vi "LSMcontroller_v56_from here for labview64bit.vi"() -> ()   [LabVIEW 2015] (continued)
                        n3651 = control-ref of="Digital Lines Plot"() -> (w455:refnum<vi>)
                        n3652 = call "Used DO lines.vi"() -> ("used DO names"=w454:string[], "used DO lines"=w453:tag[])  [unwired: 2 in]
                        n3653 = local write "Analog Used Lines"(w458) -> ()
                        n3654 = local write "Analog Used Names"(w456) -> ()
                        n3655 = local write "Digital Used Lines"(w453) -> ()
                        n3656 = local write "Digital Used Names"(w454) -> ()
                        n3657 = call "prepDOWaveplot.vi"("DigitalGraph in"=w455, "used DO names"=w454) -> ()  [unwired: 1 in]
                        n3658 = call "prepAOWaveplot.vi"("WaveformGraph in"=w457, "Analog Used Names"=w456) -> ()  [unwired: 1 in]
                      }
                    }
                  }
                  frame #4 {
                    n3659 = local read "remAO"() -> (w459:bool)
                    n3660 = case shown="True" w459 {
                      tunnel: w460 -> [_ w461]
                      frame False {
                      }
                      frame True {
                        n3661 = call "waveformparamsv2.vi"("command"="rem AO", "index"=w461) -> ()  [unwired: 3 in, 3 out]
                      }
                    }
                  }
                  frame #5 {
                    n3662 = local read "remAO"() -> (w464:bool)
                    n3663 = case shown="True" w464 {
                      tunnel: w463 -> [_ w483]
                      frame False {
                      }
                      frame True {
                        n3664 = local read "Meastab"() -> (w468:enum32{"X-Y Image", "Linescan", "Timetrace"})
                        n3665 = property on="refwf" class="Ring (strict)"() -> ("RingText.Text"=w471:string)  [unwired: 2 in, 2 out]
                        n3666 = case shown="\"Timetrace\"" w468 {
                          tunnel: [w484 w485] -> w467
                          frame "X-Y Image", Default {
                            n3667 = local read "Sampling rate"() -> (w484:dbl)
                          }
                          frame "Timetrace" {
                            n3668 = local read "srateAODOtt"() -> (w485:dbl)
                          }
                        }
                        n3669 = call "waveformsAObuffer.vi"("command"="get") -> ("AO wf out"=w480:waveform(dbl)[])  [unwired: 1 in]
                        n3670 = call "waveformsDObuffer.vi"("command"="get") -> ("DO wf out"=w477:digitalwaveform[])  [unwired: 1 in]
                        n3671 = Delete From Array(array=w480, length=1, index=w483) -> (array with subset deleted=w472:waveform(dbl)[])  [unwired: 1 out]
                        n3672 = call "correctwaveformsizetemp.vi"("new sampling frequency (Hz)"=w467, "start"=FALSE, "reference waveforms to"=w471, "Analog waveforms in"=w472, "stop"=FALSE, "Digital waveforms in"=w477) -> ("analog wf out"=w475:waveform(dbl)[], "Digital wf out"=w473:digitalwaveform[], "measpoints"=w469:i32)
                        n3673 = local write "Analog Lines Plot"(w475) -> ()
                        n3674 = call "GetNumCamFramesv2.vi"("Digital Waveform Graph"=w473) -> ("Numeric"=w474:i32)  [unwired: 10 in]
                        n3675 = local write "Digital Lines Plot"(w473) -> ()
                        n3676 = call "waveformsAObuffer.vi"("AO wf in"=w475, "command"="set") -> ()  [unwired: 1 out]
                        n3677 = call "waveformsDObuffer.vi"("DO wf in"=w473, "command"="set") -> ()  [unwired: 1 out]
                        n3678 = local read "wavdet"() -> (w470:bool)
                        n3679 = local write "Total Camera Frames"(w474) -> ()
                        n3680 = case shown="True" w470 {
                          tunnel: w469 -> [_ w486]
                          frame False {
                          }
                          frame True {
                            n3681 = local write "# of frames"(w486) -> ()
                          }
                        }
                      }
                    }
                  }
                  frame #6 {
                    w487 = FALSE ("remAO")
                    n3682 = local read "finite samples"() -> (w488:bool)
                    n3683 = local read "continuous"() -> (w489:bool)
                    n3684 = local read "wavdet"() -> (w490:bool)
                    n3685 = call "2pparameters.vi"("command"="get") -> ("params out"=w493:T12)  [unwired: 1 in]
                    n3686 = Bundle By Name(cluster=w493, "finite"=w488, "cont"=w489, "wavdet"=w490) -> (w491:T12)
                    n3687 = local write "remAO"(w487) -> ()
                    n3688 = property on="Rem AO wave" class="Bool (strict)"("Val(Sgnl)"=w487) -> ()  [unwired: 2 in, 2 out]
                    n3689 = call "2pparameters.vi"("Params in"=w491, "command"="set") -> ()  [unwired: 1 out]
                  }
                }
              }
            }
          }
          event "Add DO wave": Value Change {
            n3690 = event-data() -> ("NewVal"=w495:bool)  [unwired: 1 in, 5 out]
            n3691 = case shown="True" w495 {
              frame False {
              }
              frame True {
                n3692 = stacked-sequence {
                  seq-local: [_ _ _ _ _ w655 _ _] -> [_ _ _ _ _ _ w670 _]
                  frame #0 {
                    n3693 = local read "Measurement"() -> (w496:T5)
                    n3694 = case shown="\"X-Y-t movie\", Default" w496 {
                      frame "X-Y-t movie", Default {
                        n3695 = local read "avpp"() -> (w517:i32)
                        n3696 = local read "Angle ref"() -> (w516:dbl)
                        n3697 = local read "ROI Type"() -> (w515:u16)
                        n3698 = local read "xpixels ref"() -> (w512:i32)
                        n3699 = local read "Vx-min ref"() -> (w511:dbl)
                        n3700 = local read "Vx-max ref"() -> (w510:dbl)
                        n3701 = local read "ypixels ref"() -> (w508:i32)
                        n3702 = local read "Vy-min ref"() -> (w509:dbl)
                        n3703 = local read "Vy-max ref"() -> (w505:dbl)
                        n3704 = local read "Sampling rate"() -> (w499:dbl)
                        n3705 = local read "finite samples"() -> (w500:bool)
                        n3706 = local read "continuous"() -> (w503:bool)
                        n3707 = local read "wavdet"() -> (w504:bool)
                        n3708 = local read "# of frames"() -> (w502:i32)
                        n3709 = local read "maxbufferAI"() -> (w501:i32)
                        n3710 = local read "Override AI buffer"() -> (w497:bool)
                        n3711 = call "2pparameters.vi"("command"="get") -> ("params out"=w514:T12)  [unwired: 1 in]
                        n3712 = Bundle By Name(cluster=w514, "type"="X-Y-t movie", "avpp"=w517, "Angle Img"=w516, "Xpixels Img"=w512, "Vx-min Img"=w511, "VX-max Img"=w510, "Ypixels Img"=w508, "Vy-min Img"=w509, "Vy-max Img"=w505, "srate"=w499, "srate Img"=w499, "finite"=w500, "cont"=w503, "wavdet"=w504, "measpoints"=w502, "maxbufferAI"=w501, "Drawing Mode"=w515, "Vz-reset"=0.0, "AIoverride"=w497) -> (w506:T12)
                        n3713 = call "2pparameters.vi"("Params in"=w506, "command"="set") -> ()  [unwired: 1 out]
                      }
                      frame "X-Y-Z stack" {
                        n3714 = call "2pparameters.vi"("command"="get") -> ("params out"=w521:T12)  [unwired: 1 in]
                        n3715 = Bundle By Name(cluster=w521, "type"="X-Y-Z stack") -> (w519:T12)
                        n3716 = call "2pparameters.vi"("Params in"=w519, "command"="set") -> ()  [unwired: 1 out]
                      }
                      frame "Lifetime (scan)" {
                        n3717 = call "2pparameters.vi"("command"="get") -> ("params out"=w526:T12)  [unwired: 1 in]
                        n3718 = Bundle By Name(cluster=w526, "type"="Lifetime (scan)") -> (w524:T12)
                        n3719 = call "2pparameters.vi"("Params in"=w524, "command"="set") -> ()  [unwired: 1 out]
                      }
                      frame "Lifetime (contour)" {
                        n3720 = local read "Vy-min draw"() -> (w536:dbl)
                        n3721 = local read "Vy-max draw"() -> (w535:dbl)
                        n3722 = local read "Vx-min draw"() -> (w538:dbl)
                        n3723 = local read "Vx-max draw"() -> (w537:dbl)
                        n3724 = local read "xpixels ref"() -> (w534:i32)
                        n3725 = local read "ypixels ref"() -> (w533:i32)
                        n3726 = local read "ROI Type"() -> (w532:u16)
                        n3727 = local read "srateAODOtt"() -> (w543:dbl)
                        n3728 = local read "# of frames"() -> (w548:i32)
                        n3729 = local read "refreshtime"() -> (w540:dbl)
                        n3730 = local read "Pel"() -> (w531:dbl)
                        n3731 = local read "bin"() -> (w546:dbl)
                        n3732 = local read "Override AI buffer"() -> (w529:bool)
                        n3733 = local read "finite samples"() -> (w555:bool)
                        n3734 = local read "srateAODOtt"() -> (w542:dbl)
                        n3735 = local read "srateAODOtt"() -> (w549:dbl)
                        n3736 = local read "continuous"() -> (w554:bool)
                        n3737 = local read "Angle ref"() -> (w539:dbl)
                        n3738 = local read "wavdet"() -> (w556:bool)
                        n3739 = local read "Vx-ref"() -> (w551:dbl)
                        n3740 = local read "Vy-ref"() -> (w553:dbl)
                        n3741 = local read "avpp"() -> (w552:i32)
                        n3742 = call "tt_timeandsamples.vi"("bin"=w546, "refreshtime"=w540, "srateAODOtt"=w543, "tot#ofsamples"=w548) -> ("refreshrate"=w544:dbl, "refreshbuffer"=w545:i32, "timetracecycles"=w550:i32)  [unwired: 5 in]
                        n3743 = local read "bin"() -> (w547:dbl)
                        n3744 = call "2pparameters.vi"("command"="get") -> ("params out"=w559:T12)  [unwired: 1 in]
                        n3745 = Bundle By Name(cluster=w559, "Drawing Mode"=w532, "measpoints"=w548, "tt_cycles"=w550, "refreshbuffer"=w545, "refreshrate"=w544, "Vx-ref"=w551, "Vy-ref"=w553, "srate"=w542, "finite"=w555, "cont"=w554, "wavdet"=w556, "avpp"=w552, "srateAODO"=w549, "bufferAI"=w545, "bin"=w547, "Angle Img"=w539, "Vxminref"=w538, "Vxmaxref"=w537, "Vyminref"=w536, "Vymaxref"=w535, "Xpixels Img"=w534, "Ypixels Img"=w533, "Pel"=w531, "Vz-reset"=0.0, "AIoverride"=w529, "type"="Lifetime (contour)") -> (w557:T12)
                        n3746 = Reciprocal(x=w544) -> (1/x=w541:dbl)
                        n3747 = local write "refreshtime"(w541) -> ()
                        n3748 = call "2pparameters.vi"("Params in"=w557, "command"="set") -> ()  [unwired: 1 out]
                      }
                      frame "X-Y-Z-t movie" {
                      }
                      frame "linescan" {
                      }
                      frame "Timetrace" {
                        n3749 = local read "Vy-min draw"() -> (w569:dbl)
                        n3750 = local read "Vy-max draw"() -> (w568:dbl)
                        n3751 = local read "Vx-min draw"() -> (w571:dbl)
                        n3752 = local read "Vx-max draw"() -> (w570:dbl)
                        n3753 = local read "xpixels ref"() -> (w567:i32)
                        n3754 = local read "ypixels ref"() -> (w566:i32)
                        n3755 = local read "ROI Type"() -> (w565:u16)
                        n3756 = local read "srateAODOtt"() -> (w576:dbl)
                        n3757 = local read "# of frames"() -> (w581:i32)
                        n3758 = local read "refreshtime"() -> (w573:dbl)
                        n3759 = local read "Pel"() -> (w564:dbl)
                        n3760 = local read "bin"() -> (w579:dbl)
                        n3761 = local read "Override AI buffer"() -> (w562:bool)
                        n3762 = local read "finite samples"() -> (w588:bool)
                        n3763 = local read "srateAODOtt"() -> (w575:dbl)
                        n3764 = local read "srateAODOtt"() -> (w582:dbl)
                        n3765 = local read "continuous"() -> (w587:bool)
                        n3766 = local read "Angle ref"() -> (w572:dbl)
                        n3767 = local read "wavdet"() -> (w589:bool)
                        n3768 = local read "Vx-ref"() -> (w584:dbl)
                        n3769 = local read "Vy-ref"() -> (w586:dbl)
                        n3770 = local read "avpp"() -> (w585:i32)
                        n3771 = call "tt_timeandsamples.vi"("bin"=w579, "refreshtime"=w573, "srateAODOtt"=w576, "tot#ofsamples"=w581) -> ("refreshrate"=w577:dbl, "refreshbuffer"=w578:i32, "timetracecycles"=w583:i32)  [unwired: 5 in]
                        n3772 = local read "bin"() -> (w580:dbl)
                        n3773 = call "2pparameters.vi"("command"="get") -> ("params out"=w592:T12)  [unwired: 1 in]
                        n3774 = Bundle By Name(cluster=w592, "Drawing Mode"=w565, "measpoints"=w581, "tt_cycles"=w583, "refreshbuffer"=w578, "refreshrate"=w577, "Vx-ref"=w584, "Vy-ref"=w586, "srate"=w575, "finite"=w588, "cont"=w587, "wavdet"=w589, "avpp"=w585, "srateAODO"=w582, "bufferAI"=w578, "bin"=w580, "Angle Img"=w572, "Vxminref"=w571, "Vxmaxref"=w570, "Vyminref"=w569, "Vymaxref"=w568, "Xpixels Img"=w567, "Ypixels Img"=w566, "Pel"=w564, "Vz-reset"=0.0, "AIoverride"=w562, "type"="Timetrace") -> (w590:T12)
                        n3775 = Reciprocal(x=w577) -> (1/x=w574:dbl)
                        n3776 = local write "refreshtime"(w574) -> ()
                        n3777 = call "2pparameters.vi"("Params in"=w590, "command"="set") -> ()  [unwired: 1 out]
                      }
                      frame "Lifetime (point)" {
                      }
                    }
                  }
                  frame #1 {
                    w595 = FALSE ("wavdet")
                    n3778 = call "2pparameters.vi"("command"="get") -> ("params out"=w599:T12)  [unwired: 1 in]
                    n3779 = Bundle By Name(cluster=w599, "finite"=w595, "cont"=w595, "wavdet"=TRUE) -> (w596:T12)
                    n3780 = call "2pparameters.vi"("Params in"=w596, "command"="set") -> ()  [unwired: 1 out]
                  }
                  frame #2 {
                    n3781 = local read "DO channels"() -> (w606:u16)
                    n3782 = call "2pparameters.vi"("command"="get") -> ("params out"=w604:T12)  [unwired: 1 in]
                    n3783 = in-place {
                      in-place-border: w606 -> [w610]
                      in-place-border: [w607] -> w601
                      n3784 = in-place-cluster #51(w604) -> ("aDO"=w609:u32[])
                      n3785 = call "add channel to active arrayv2.vi"("line array in"=w609, "line to add"=w610) -> ("line array out"=w608:u32[], "addition"=w607:bool)  [unwired: 1 out]
                      n3786 = in-place-cluster #51("aDO"=w608) -> (w602:T12)
                    }
                    n3787 = local write "addDO"(w601) -> ()
                    n3788 = call "2pparameters.vi"("Params in"=w602, "command"="set") -> ()  [unwired: 1 out]
                  }
                  frame #3 {
                    n3789 = local read "addDO"() -> (w611:bool)
                    n3790 = case shown="True" w611 {
                      frame False {
                      }
                      frame True {
                        n3791 = call "Used AO lines.vi"() -> ("used AO names"=w615:string[], "used AO lines"=w617:tag[])  [unwired: 2 in]
                        n3792 = control-ref of="Analog Lines Plot"() -> (w616:refnum<vi>)
                        n3793 = control-ref of="Digital Lines Plot"() -> (w614:refnum<vi>)
                        n3794 = call "Used DO lines.vi"() -> ("used DO names"=w613:string[], "used DO lines"=w612:tag[])  [unwired: 2 in]
                        n3795 = local write "Analog Used Lines"(w617) -> ()
                        n3796 = local write "Analog Used Names"(w615) -> ()
                        n3797 = local write "Digital Used Lines"(w612) -> ()
                        n3798 = local write "Digital Used Names"(w613) -> ()
                        n3799 = call "prepDOWaveplot.vi"("DigitalGraph in"=w614, "used DO names"=w613) -> ()  [unwired: 1 in]
                        n3800 = call "prepAOWaveplot.vi"("WaveformGraph in"=w616, "Analog Used Names"=w615) -> ()  [unwired: 1 in]
                      }
                    }
                  }
                  frame #4 {
                    n3801 = local read "addDO"() -> (w618:bool)
                    n3802 = case shown="True" w618 {
                      frame False {
                      }
                      frame True {
                        n3803 = local read "Build digital waveform tabs"() -> (w619:enum32{"Simple", "Matlab"})
                        n3804 = case shown="\"Matlab\"" w619 {
                          frame "Simple", Default {
                            n3805 = local read "Meastab"() -> (w621:enum32{"X-Y Image", "Linescan", "Timetrace"})
                            n3806 = call "waveformparamsv2.vi"("command"="get") -> ("Params out"=w635:T16)  [unwired: 4 in, 2 out]
                            n3807 = case shown="\"Timetrace\"" w621 {
                              tunnel: [w637 w638] -> w620
                              frame "X-Y Image", Default {
                                n3808 = local read "Sampling rate"() -> (w637:dbl)
                              }
                              frame "Timetrace" {
                                n3809 = local read "srateAODOtt"() -> (w638:dbl)
                              }
                            }
                            n3810 = Unbundle By Name(w635) -> ("DO parameters"=w633:T19)
                            n3811 = local read "Digital padding value"() -> (w624:dbl)
                            n3812 = local read "Digital time offset (s)"() -> (w625:dbl)
                            n3813 = local read "Digital phase (s)"() -> (w627:dbl)
                            n3814 = local read "Digital Freq (Hz)"() -> (w626:dbl)
                            n3815 = local read "Digital DC (%)"() -> (w628:dbl)
                            n3816 = Index Array(array=w633, index=0) -> (element=w632:T20)
                            n3817 = Bundle By Name(cluster=w632, "Digital DC (%)"=w628, "Digital phase"=w627, "Digital Freq (Hz)"=w626, "Sampling frequency (Hz)"=w620, "Digital time offset (s)"=w625, "padding value"=w624, "matlab wave file"=path "", "DOtab"=0.0) -> (w630:T20)
                            n3818 = Build Array(w630) -> (w629:T19)
                            n3819 = call "waveformparamsv2.vi"("command"="add DO", "add DO"=w629) -> ()  [unwired: 3 in, 3 out]
                          }
                          frame "Matlab" {
                            w642 = 0.0 ("DOtab")
                            n3820 = local read "Meastab"() -> (w640:enum32{"X-Y Image", "Linescan", "Timetrace"})
                            n3821 = call "waveformparamsv2.vi"("command"="get") -> ("Params out"=w651:T16)  [unwired: 4 in, 2 out]
                            n3822 = case shown="\"Timetrace\"" w640 {
                              tunnel: [w653 w654] -> w639
                              frame "X-Y Image", Default {
                                n3823 = local read "Sampling rate"() -> (w653:dbl)
                              }
                              frame "Timetrace" {
                                n3824 = local read "srateAODOtt"() -> (w654:dbl)
                              }
                            }
                            n3825 = Unbundle By Name(w651) -> ("DO parameters"=w649:T19)
                            n3826 = local read "Matlab waveform path DO"() -> (w641:path)
                            n3827 = local read "Matlab padding value DO"() -> (w644:dbl)
                            n3828 = Index Array(array=w649, index=0) -> (element=w648:T20)
                            n3829 = Bundle By Name(cluster=w648, "Digital DC (%)"=w642, "Digital phase"=w642, "Digital Freq (Hz)"=w642, "Sampling frequency (Hz)"=w639, "Digital time offset (s)"=w642, "padding value"=w644, "matlab wave file"=w641, "DOtab"=1.0) -> (w646:T20)
                            n3830 = Build Array(w646) -> (w645:T19)
                            n3831 = call "waveformparamsv2.vi"("command"="add DO", "add DO"=w645) -> ()  [unwired: 3 in, 3 out]
                          }
                        }
                      }
                    }
                  }
                  frame #5 {
                    n3832 = local read "addDO"() -> (w656:bool)
                    n3833 = case shown="True" w656 {
                      tunnel: [_ w657] -> w655
                      frame False {
                      }
                      frame True {
                        n3834 = property on="refwf" class="Ring (strict)"() -> ("RingText.Text"=w662:string)  [unwired: 2 in, 2 out]
                        n3835 = call "waveformsDObuffer.vi"("command"="get") -> ("DO wf out"=w661:digitalwaveform[])  [unwired: 1 in]
                        n3836 = call "waveformsAObuffer.vi"("command"="get") -> ("AO wf out"=w659:waveform(dbl)[])  [unwired: 1 in]
                        n3837 = call "referfencesize.vi"("Digital waveforms in"=w661, "Analog waveforms in"=w659, "reference waveforms to"=w662) -> ("number of samples"=w657:i32)  [unwired: 2 in]
                      }
                    }
                  }
                  frame #6 {
                    n3838 = local read "Build digital waveform tabs"() -> (w673:enum32{"Simple", "Matlab"})
                    n3839 = call "waveformparamsv2.vi"("command"="get last DO") -> ("last DO"=w672:T20)  [unwired: 4 in, 2 out]
                    n3840 = local read "Meastab"() -> (w666:enum32{"X-Y Image", "Linescan", "Timetrace"})
                    n3841 = call "waveformsDObuffer.vi"("command"="get") -> ("DO wf out"=w671:digitalwaveform[])  [unwired: 1 in]
                    n3842 = case shown="\"Simple\", Default" w673 {
                      tunnel: w672 -> [w690 w692]
                      tunnel: w670 -> [w689 _]
                      tunnel: [w688 w691] -> w669
                      frame "Simple", Default {
                        n3843 = call "simple digital from wf params.vi"("waveform params"=w690, "number of samples"=w689) -> ("digital waveform"=w688:digitalwaveform)
                      }
                      frame "Matlab" {
                        n3844 = call "matlabDOwffromparam.vi"("waveform params"=w692) -> ("digital waveform"=w691:digitalwaveform)
                      }
                    }
                    n3845 = property on="refwf" class="Ring (strict)"() -> ("RingText.Text"=w676:string)  [unwired: 2 in, 2 out]
                    n3846 = case shown="\"Timetrace\"" w666 {
                      tunnel: [w685 w686] -> w665
                      frame "X-Y Image", Default {
                        n3847 = local read "Sampling rate"() -> (w685:dbl)
                      }
                      frame "Timetrace" {
                        n3848 = local read "srateAODOtt"() -> (w686:dbl)
                      }
                    }
                    n3849 = call "waveformsAObuffer.vi"("command"="get") -> ("AO wf out"=w684:waveform(dbl)[])  [unwired: 1 in]
                    n3850 = Build Array (concatenate)(w671, w669) -> (w675:digitalwaveform[])
                    n3851 = call "correctwaveformsizetemp.vi"("new sampling frequency (Hz)"=w665, "start"=FALSE, "reference waveforms to"=w676, "Analog waveforms in"=w684, "stop"=FALSE, "Digital waveforms in"=w675) -> ("analog wf out"=w679:waveform(dbl)[], "Digital wf out"=w677:digitalwaveform[], "measpoints"=w667:i32)
                    n3852 = local write "Analog Lines Plot"(w679) -> ()
                    n3853 = call "GetNumCamFramesv2.vi"("Digital Waveform Graph"=w677) -> ("Numeric"=w678:i32)  [unwired: 10 in]
                    n3854 = local write "Digital Lines Plot"(w677) -> ()
                    n3855 = call "waveformsAObuffer.vi"("AO wf in"=w679, "command"="set") -> ()  [unwired: 1 out]
                    n3856 = call "waveformsDObuffer.vi"("DO wf in"=w677, "command"="set") -> ()  [unwired: 1 out]
                    n3857 = local write "Total Camera Frames"(w678) -> ()
                    n3858 = local read "wavdet"() -> (w668:bool)
                    n3859 = case shown="True" w668 {
                      tunnel: w667 -> [_ w687]
                      frame False {
                      }
                      frame True {
                        n3860 = local write "# of frames"(w687) -> ()
                      }
                    }
                  }
                  frame #7 {
                    w693 = FALSE ("addAO")
                    n3861 = local read "finite samples"() -> (w694:bool)
                    n3862 = local read "continuous"() -> (w695:bool)
                    n3863 = local read "wavdet"() -> (w696:bool)
                    n3864 = call "2pparameters.vi"("command"="get") -> ("params out"=w699:T12)  [unwired: 1 in]
                    n3865 = Bundle By Name(cluster=w699, "finite"=w694, "cont"=w695, "wavdet"=w696) -> (w697:T12)
                    n3866 = call "2pparameters.vi"("Params in"=w697, "command"="set") -> ()  [unwired: 1 out]
                    n3867 = local write "addDO"(w693) -> ()
                    n3868 = property on="Add DO wave" class="Bool (strict)"("Val(Sgnl)"=w693) -> ()  [unwired: 2 in, 2 out]
                  }
                }
              }
            }
          }
          event "DO channels": Value Change {
            n3869 = event-data() -> ()  [unwired: 1 in, 6 out]
            n3870 = local read "DO channels"() -> (w703:u16)
            n3871 = call "2pparameters.vi"("command"="get") -> ("params out"=w705:T12)  [unwired: 1 in]
            n3872 = Unbundle By Name(w705) -> ("aDO"=w704:u32[])
            n3873 = Search 1D Array(1D array=w704, element=w703) -> (index of element=w702:i32)  [unwired: 1 in]
            n3874 = Equal?(x=w702, y=-1.0) -> (x = y?=w701:bool)
            n3875 = case shown="False" w701 {
              tunnel: w702 -> [w720 _]
              frame False {
                n3876 = call "waveformparamsv2.vi"("command"="get") -> ("Params out"=w715:T16)  [unwired: 4 in, 2 out]
                n3877 = Unbundle By Name(w715) -> ("DO parameters"=w713:T19)
                n3878 = Index Array(array=w713, index=w720) -> (element=w719:T20)
                n3879 = Unbundle By Name(w719) -> ("Digital DC (%)"=w718:dbl, "Digital phase"=w717:dbl, "Digital Freq (Hz)"=w716:dbl, "Sampling frequency (Hz)"=w708:dbl, "Digital time offset (s)"=w712:dbl, "padding value"=w711:dbl, "matlab wave file"=w710:path, "DOtab"=w709:dbl)
                n3880 = local write "Build digital waveform tabs"(w709) -> ()
                n3881 = local write "Digital DC (%)"(w718) -> ()
                n3882 = local write "Matlab waveform path DO"(w710) -> ()
                n3883 = local write "Digital time offset (s)"(w712) -> ()
                n3884 = local write "Matlab padding value DO"(w711) -> ()
                n3885 = local write "Digital padding value"(w711) -> ()
                n3886 = local write "Sampling rate \ncurrent wf"(w708) -> ()
                n3887 = local write "Digital Freq (Hz)"(w716) -> ()
                n3888 = local write "Digital phase (s)"(w717) -> ()
              }
              frame True {
              }
            }
          }
          event "Rem DO wave": Value Change {
            n3889 = event-data() -> ("NewVal"=w721:bool)  [unwired: 1 in, 5 out]
            n3890 = case shown="True" w721 {
              frame False {
              }
              frame True {
                n3891 = stacked-sequence {
                  seq-local: [_ _ w827 _ _ _ _] -> [_ _ _ _ w846 w857 _]
                  frame #0 {
                    n3892 = local read "Measurement"() -> (w722:T5)
                    n3893 = case shown="\"linescan\"" w722 {
                      frame "X-Y-t movie", Default {
                        n3894 = local read "avpp"() -> (w743:i32)
                        n3895 = local read "Angle ref"() -> (w742:dbl)
                        n3896 = local read "ROI Type"() -> (w741:u16)
                        n3897 = local read "xpixels ref"() -> (w738:i32)
                        n3898 = local read "Vx-min ref"() -> (w737:dbl)
                        n3899 = local read "Vx-max ref"() -> (w736:dbl)
                        n3900 = local read "ypixels ref"() -> (w734:i32)
                        n3901 = local read "Vy-min ref"() -> (w735:dbl)
                        n3902 = local read "Vy-max ref"() -> (w731:dbl)
                        n3903 = local read "Sampling rate"() -> (w725:dbl)
                        n3904 = local read "finite samples"() -> (w726:bool)
                        n3905 = local read "continuous"() -> (w729:bool)
                        n3906 = local read "wavdet"() -> (w730:bool)
                        n3907 = local read "# of frames"() -> (w728:i32)
                        n3908 = local read "maxbufferAI"() -> (w727:i32)
                        n3909 = local read "Override AI buffer"() -> (w723:bool)
                        n3910 = call "2pparameters.vi"("command"="get") -> ("params out"=w740:T12)  [unwired: 1 in]
                        n3911 = Bundle By Name(cluster=w740, "type"="X-Y-t movie", "avpp"=w743, "Angle Img"=w742, "Xpixels Img"=w738, "Vx-min Img"=w737, "VX-max Img"=w736, "Ypixels Img"=w734, "Vy-min Img"=w735, "Vy-max Img"=w731, "srate"=w725, "srate Img"=w725, "finite"=w726, "cont"=w729, "wavdet"=w730, "measpoints"=w728, "maxbufferAI"=w727, "Drawing Mode"=w741, "Vz-reset"=0.0, "AIoverride"=w723) -> (w732:T12)
                        n3912 = call "2pparameters.vi"("Params in"=w732, "command"="set") -> ()  [unwired: 1 out]
                      }
                      frame "X-Y-Z stack" {
                        n3913 = call "2pparameters.vi"("command"="get") -> ("params out"=w747:T12)  [unwired: 1 in]
                        n3914 = Bundle By Name(cluster=w747, "type"="X-Y-Z stack") -> (w745:T12)
                        n3915 = call "2pparameters.vi"("Params in"=w745, "command"="set") -> ()  [unwired: 1 out]
                      }
                      frame "Lifetime (scan)" {
                        n3916 = call "2pparameters.vi"("command"="get") -> ("params out"=w752:T12)  [unwired: 1 in]
                        n3917 = Bundle By Name(cluster=w752, "type"="Lifetime (scan)") -> (w750:T12)
                        n3918 = call "2pparameters.vi"("Params in"=w750, "command"="set") -> ()  [unwired: 1 out]
                      }
                      frame "Lifetime (contour)" {
                        n3919 = local read "Vy-min draw"() -> (w762:dbl)
                        n3920 = local read "Vy-max draw"() -> (w761:dbl)
                        n3921 = local read "Vx-min draw"() -> (w764:dbl)
                        n3922 = local read "Vx-max draw"() -> (w763:dbl)
                        n3923 = local read "xpixels ref"() -> (w760:i32)
                        n3924 = local read "ypixels ref"() -> (w759:i32)
                        n3925 = local read "ROI Type"() -> (w758:u16)
                        n3926 = local read "srateAODOtt"() -> (w769:dbl)
                        n3927 = local read "# of frames"() -> (w774:i32)
                        n3928 = local read "refreshtime"() -> (w766:dbl)
                        n3929 = local read "Pel"() -> (w757:dbl)
                        n3930 = local read "bin"() -> (w772:dbl)
                        n3931 = local read "Override AI buffer"() -> (w755:bool)
                        n3932 = local read "finite samples"() -> (w781:bool)
                        n3933 = local read "srateAODOtt"() -> (w768:dbl)
                        n3934 = local read "srateAODOtt"() -> (w775:dbl)
                        n3935 = local read "continuous"() -> (w780:bool)
                        n3936 = local read "Angle ref"() -> (w765:dbl)
                        n3937 = local read "wavdet"() -> (w782:bool)
                        n3938 = local read "Vx-ref"() -> (w777:dbl)
                        n3939 = local read "Vy-ref"() -> (w779:dbl)
                        n3940 = local read "avpp"() -> (w778:i32)
                        n3941 = call "tt_timeandsamples.vi"("bin"=w772, "refreshtime"=w766, "srateAODOtt"=w769, "tot#ofsamples"=w774) -> ("refreshrate"=w770:dbl, "refreshbuffer"=w771:i32, "timetracecycles"=w776:i32)  [unwired: 5 in]
                        n3942 = local read "bin"() -> (w773:dbl)
                        n3943 = call "2pparameters.vi"("command"="get") -> ("params out"=w785:T12)  [unwired: 1 in]
                        n3944 = Bundle By Name(cluster=w785, "Drawing Mode"=w758, "measpoints"=w774, "tt_cycles"=w776, "refreshbuffer"=w771, "refreshrate"=w770, "Vx-ref"=w777, "Vy-ref"=w779, "srate"=w768, "finite"=w781, "cont"=w780, "wavdet"=w782, "avpp"=w778, "srateAODO"=w775, "bufferAI"=w771, "bin"=w773, "Angle Img"=w765, "Vxminref"=w764, "Vxmaxref"=w763, "Vyminref"=w762, "Vymaxref"=w761, "Xpixels Img"=w760, "Ypixels Img"=w759, "Pel"=w757, "Vz-reset"=0.0, "AIoverride"=w755, "type"="Lifetime (contour)") -> (w783:T12)
                        n3945 = Reciprocal(x=w770) -> (1/x=w767:dbl)
                        n3946 = local write "refreshtime"(w767) -> ()
                        n3947 = call "2pparameters.vi"("Params in"=w783, "command"="set") -> ()  [unwired: 1 out]
                      }
                      frame "X-Y-Z-t movie" {
                      }
                      frame "linescan" {
                      }
                      frame "Timetrace" {
                        n3948 = local read "Vy-min draw"() -> (w795:dbl)
                        n3949 = local read "Vy-max draw"() -> (w794:dbl)
                        n3950 = local read "Vx-min draw"() -> (w797:dbl)
                        n3951 = local read "Vx-max draw"() -> (w796:dbl)
                        n3952 = local read "xpixels ref"() -> (w793:i32)
                        n3953 = local read "ypixels ref"() -> (w792:i32)
                        n3954 = local read "ROI Type"() -> (w791:u16)
                        n3955 = local read "srateAODOtt"() -> (w802:dbl)
                        n3956 = local read "# of frames"() -> (w807:i32)
                        n3957 = local read "refreshtime"() -> (w799:dbl)
                        n3958 = local read "Pel"() -> (w790:dbl)
                        n3959 = local read "bin"() -> (w805:dbl)
                        n3960 = local read "Override AI buffer"() -> (w788:bool)
                        n3961 = local read "finite samples"() -> (w814:bool)
                        n3962 = local read "srateAODOtt"() -> (w801:dbl)
                        n3963 = local read "srateAODOtt"() -> (w808:dbl)
                        n3964 = local read "continuous"() -> (w813:bool)
                        n3965 = local read "Angle ref"() -> (w798:dbl)
                        n3966 = local read "wavdet"() -> (w815:bool)
                        n3967 = local read "Vx-ref"() -> (w810:dbl)
                        n3968 = local read "Vy-ref"() -> (w812:dbl)
                        n3969 = local read "avpp"() -> (w811:i32)
                        n3970 = call "tt_timeandsamples.vi"("bin"=w805, "refreshtime"=w799, "srateAODOtt"=w802, "tot#ofsamples"=w807) -> ("refreshrate"=w803:dbl, "refreshbuffer"=w804:i32, "timetracecycles"=w809:i32)  [unwired: 5 in]
                        n3971 = local read "bin"() -> (w806:dbl)
                        n3972 = call "2pparameters.vi"("command"="get") -> ("params out"=w818:T12)  [unwired: 1 in]
                        n3973 = Bundle By Name(cluster=w818, "Drawing Mode"=w791, "measpoints"=w807, "tt_cycles"=w809, "refreshbuffer"=w804, "refreshrate"=w803, "Vx-ref"=w810, "Vy-ref"=w812, "srate"=w801, "finite"=w814, "cont"=w813, "wavdet"=w815, "avpp"=w811, "srateAODO"=w808, "bufferAI"=w804, "bin"=w806, "Angle Img"=w798, "Vxminref"=w797, "Vxmaxref"=w796, "Vyminref"=w795, "Vymaxref"=w794, "Xpixels Img"=w793, "Ypixels Img"=w792, "Pel"=w790, "Vz-reset"=0.0, "AIoverride"=w788, "type"="Timetrace") -> (w816:T12)
                        n3974 = Reciprocal(x=w803) -> (1/x=w800:dbl)
                        n3975 = local write "refreshtime"(w800) -> ()
                        n3976 = call "2pparameters.vi"("Params in"=w816, "command"="set") -> ()  [unwired: 1 out]
                      }
                      frame "Lifetime (point)" {
                      }
                    }
                  }
                  frame #1 {
                    w821 = FALSE ("wavdet")
                    n3977 = call "2pparameters.vi"("command"="get") -> ("params out"=w825:T12)  [unwired: 1 in]
                    n3978 = Bundle By Name(cluster=w825, "finite"=w821, "cont"=w821, "wavdet"=TRUE) -> (w822:T12)
                    n3979 = call "2pparameters.vi"("Params in"=w822, "command"="set") -> ()  [unwired: 1 out]
                  }
                  frame #2 {
                    n3980 = local read "DO channels"() -> (w833:u16)
                    n3981 = call "2pparameters.vi"("command"="get") -> ("params out"=w831:T12)  [unwired: 1 in]
                    n3982 = in-place {
                      in-place-border: w833 -> [w838]
                      in-place-border: [w835] -> w828
                      in-place-border: [w834] -> w827
                      n3983 = in-place-cluster #52(w831) -> ("aDO"=w837:u32[])
                      n3984 = call "remove channel from active arrayv2.vi"("line array in"=w837, "line to remove"=w838) -> ("line array out"=w836:u32[], "removal"=w835:bool, "index"=w834:i32)
                      n3985 = in-place-cluster #52("aDO"=w836) -> (w829:T12)
                    }
                    n3986 = local write "remDO"(w828) -> ()
                    n3987 = call "2pparameters.vi"("Params in"=w829, "command"="set") -> ()  [unwired: 1 out]
                  }
                  frame #3 {
                    n3988 = local read "remDO"() -> (w839:bool)
                    n3989 = case shown="True" w839 {
                      frame False {
                      }
                      frame True {
                        n3990 = call "Used AO lines.vi"() -> ("used AO names"=w843:string[], "used AO lines"=w845:tag[])  [unwired: 2 in]
                        n3991 = local write "Analog Used Lines"(w845) -> ()
                        n3992 = local write "Analog Used Names"(w843) -> ()
                        n3993 = call "Used DO lines.vi"() -> ("used DO names"=w841:string[], "used DO lines"=w840:tag[])  [unwired: 2 in]
                        n3994 = control-ref of="Analog Lines Plot"() -> (w844:refnum<vi>)
                        n3995 = control-ref of="Digital Lines Plot"() -> (w842:refnum<vi>)
                        n3996 = local write "Digital Used Lines"(w840) -> ()
                        n3997 = local write "Digital Used Names"(w841) -> ()
                        n3998 = call "prepAOWaveplot.vi"("WaveformGraph in"=w844, "Analog Used Names"=w843) -> ()  [unwired: 1 in]
                        n3999 = call "prepDOWaveplot.vi"("DigitalGraph in"=w842, "used DO names"=w841) -> ()  [unwired: 1 in]
                      }
                    }
                  }
                  frame #4 {
                    n4000 = local read "remDO"() -> (w847:bool)
                    n4001 = case shown="True" w847 {
                      tunnel: w846 -> [_ w848]
                      frame False {
                      }
                      frame True {
                        n4002 = call "waveformparamsv2.vi"("command"="rem DO", "index"=w848) -> ()  [unwired: 3 in, 3 out]
                      }
                    }
                  }
                  frame #5 {
                    n4003 = local read "Meastab"() -> (w853:enum32{"X-Y Image", "Linescan", "Timetrace"})
                    n4004 = property on="refwf" class="Ring (strict)"() -> ("RingText.Text"=w860:string)  [unwired: 2 in, 2 out]
                    n4005 = call "waveformsDObuffer.vi"("command"="get") -> ("DO wf out"=w859:digitalwaveform[])  [unwired: 1 in]
                    n4006 = case shown="\"Timetrace\"" w853 {
                      tunnel: [w869 w870] -> w852
                      frame "X-Y Image", Default {
                        n4007 = local read "Sampling rate"() -> (w869:dbl)
                      }
                      frame "Timetrace" {
                        n4008 = local read "srateAODOtt"() -> (w870:dbl)
                      }
                    }
                    n4009 = call "waveformsAObuffer.vi"("command"="get") -> ("AO wf out"=w868:waveform(dbl)[])  [unwired: 1 in]
                    n4010 = Delete From Array(array=w859, length=1, index=w857) -> (array with subset deleted=w856:digitalwaveform[])  [unwired: 1 out]
                    n4011 = call "correctwaveformsizetemp.vi"("new sampling frequency (Hz)"=w852, "start"=FALSE, "reference waveforms to"=w860, "Analog waveforms in"=w868, "stop"=FALSE, "Digital waveforms in"=w856) -> ("analog wf out"=w863:waveform(dbl)[], "Digital wf out"=w861:digitalwaveform[], "measpoints"=w854:i32)
                    n4012 = local read "wavdet"() -> (w855:bool)
                    n4013 = call "waveformsAObuffer.vi"("AO wf in"=w863, "command"="set") -> ()  [unwired: 1 out]
                    n4014 = call "waveformsDObuffer.vi"("DO wf in"=w861, "command"="set") -> ()  [unwired: 1 out]
                    n4015 = local write "Analog Lines Plot"(w863) -> ()
                    n4016 = local write "Digital Lines Plot"(w861) -> ()
                    n4017 = call "GetNumCamFramesv2.vi"("Digital Waveform Graph"=w861) -> ("Numeric"=w862:i32)  [unwired: 10 in]
                    n4018 = case shown="True" w855 {
                      tunnel: w854 -> [_ w871]
                      frame False {
                      }
                      frame True {
                        n4019 = local write "# of frames"(w871) -> ()
                      }
                    }
                    n4020 = local write "Total Camera Frames"(w862) -> ()
                  }
                  frame #6 {
                    w872 = FALSE ("addAO")
                    n4021 = local read "finite samples"() -> (w873:bool)
                    n4022 = local read "continuous"() -> (w874:bool)
                    n4023 = local read "wavdet"() -> (w875:bool)
                    n4024 = local write "remDO"(w872) -> ()
                    n4025 = call "2pparameters.vi"("command"="get") -> ("params out"=w878:T12)  [unwired: 1 in]
                    n4026 = Bundle By Name(cluster=w878, "finite"=w873, "cont"=w874, "wavdet"=w875) -> (w876:T12)
                    n4027 = property on="Rem DO wave" class="Bool (strict)"("Val(Sgnl)"=w872) -> ()  [unwired: 2 in, 2 out]
                    n4028 = call "2pparameters.vi"("Params in"=w876, "command"="set") -> ()  [unwired: 1 out]
                  }
                }
              }
            }
          }
          event "Digital phase (s)", "Digital DC (%)", "Digital Freq (Hz)", "Digital padding value", "Digital time offset (s)": Value Change {
            n4029 = event-data() -> ()  [unwired: 1 in, 6 out]
            n4030 = stacked-sequence {
              seq-local: [_ _ w986 _ _] -> [_ _ _ w1003 _]
              seq-local: [_ _ w985 _ _] -> [_ _ _ w1002 _]
              frame #0 {
                n4031 = local read "Measurement"() -> (w880:T5)
                n4032 = case shown="\"X-Y-t movie\", Default" w880 {
                  frame "X-Y-t movie", Default {
                    n4033 = local read "avpp"() -> (w901:i32)
                    n4034 = local read "Angle ref"() -> (w900:dbl)
                    n4035 = local read "ROI Type"() -> (w899:u16)
                    n4036 = local read "xpixels ref"() -> (w896:i32)
                    n4037 = local read "Vx-min ref"() -> (w895:dbl)
                    n4038 = local read "Vx-max ref"() -> (w894:dbl)
                    n4039 = local read "ypixels ref"() -> (w892:i32)
                    n4040 = local read "Vy-min ref"() -> (w893:dbl)
                    n4041 = local read "Vy-max ref"() -> (w889:dbl)
                    n4042 = local read "Sampling rate"() -> (w883:dbl)
                    n4043 = local read "finite samples"() -> (w884:bool)
                    n4044 = local read "continuous"() -> (w887:bool)
                    n4045 = local read "wavdet"() -> (w888:bool)
                    n4046 = local read "# of frames"() -> (w886:i32)
                    n4047 = local read "maxbufferAI"() -> (w885:i32)
                    n4048 = local read "Override AI buffer"() -> (w881:bool)
                    n4049 = call "2pparameters.vi"("command"="get") -> ("params out"=w898:T12)  [unwired: 1 in]
                    n4050 = Bundle By Name(cluster=w898, "type"="X-Y-t movie", "avpp"=w901, "Angle Img"=w900, "Xpixels Img"=w896, "Vx-min Img"=w895, "VX-max Img"=w894, "Ypixels Img"=w892, "Vy-min Img"=w893, "Vy-max Img"=w889, "srate"=w883, "srate Img"=w883, "finite"=w884, "cont"=w887, "wavdet"=w888, "measpoints"=w886, "maxbufferAI"=w885, "Drawing Mode"=w899, "Vz-reset"=0.0, "AIoverride"=w881) -> (w890:T12)
                    n4051 = call "2pparameters.vi"("Params in"=w890, "command"="set") -> ()  [unwired: 1 out]
                  }
                  frame "X-Y-Z stack" {
                    n4052 = call "2pparameters.vi"("command"="get") -> ("params out"=w905:T12)  [unwired: 1 in]
                    n4053 = Bundle By Name(cluster=w905, "type"="X-Y-Z stack") -> (w903:T12)
                    n4054 = call "2pparameters.vi"("Params in"=w903, "command"="set") -> ()  [unwired: 1 out]
                  }
                  frame "Lifetime (scan)" {
                    n4055 = call "2pparameters.vi"("command"="get") -> ("params out"=w910:T12)  [unwired: 1 in]
                    n4056 = Bundle By Name(cluster=w910, "type"="Lifetime (scan)") -> (w908:T12)
                    n4057 = call "2pparameters.vi"("Params in"=w908, "command"="set") -> ()  [unwired: 1 out]
                  }
                  frame "Lifetime (contour)" {
                    n4058 = local read "Vy-min draw"() -> (w920:dbl)
                    n4059 = local read "Vy-max draw"() -> (w919:dbl)
                    n4060 = local read "Vx-min draw"() -> (w922:dbl)
                    n4061 = local read "Vx-max draw"() -> (w921:dbl)
                    n4062 = local read "xpixels ref"() -> (w918:i32)
                    n4063 = local read "ypixels ref"() -> (w917:i32)
                    n4064 = local read "ROI Type"() -> (w916:u16)
                    n4065 = local read "srateAODOtt"() -> (w927:dbl)
                    n4066 = local read "# of frames"() -> (w932:i32)
                    n4067 = local read "refreshtime"() -> (w924:dbl)
                    n4068 = local read "Pel"() -> (w915:dbl)
                    n4069 = local read "bin"() -> (w930:dbl)
                    n4070 = local read "Override AI buffer"() -> (w913:bool)
                    n4071 = local read "finite samples"() -> (w939:bool)
                    n4072 = local read "srateAODOtt"() -> (w926:dbl)
                    n4073 = local read "srateAODOtt"() -> (w933:dbl)
                    n4074 = local read "continuous"() -> (w938:bool)
                    n4075 = local read "Angle ref"() -> (w923:dbl)
                    n4076 = local read "wavdet"() -> (w940:bool)
                    n4077 = local read "Vx-ref"() -> (w935:dbl)
                    n4078 = local read "Vy-ref"() -> (w937:dbl)
                    n4079 = local read "avpp"() -> (w936:i32)
                    n4080 = call "tt_timeandsamples.vi"("bin"=w930, "refreshtime"=w924, "srateAODOtt"=w927, "tot#ofsamples"=w932) -> ("refreshrate"=w928:dbl, "refreshbuffer"=w929:i32, "timetracecycles"=w934:i32)  [unwired: 5 in]
                    n4081 = local read "bin"() -> (w931:dbl)
                    n4082 = call "2pparameters.vi"("command"="get") -> ("params out"=w943:T12)  [unwired: 1 in]
                    n4083 = Bundle By Name(cluster=w943, "Drawing Mode"=w916, "measpoints"=w932, "tt_cycles"=w934, "refreshbuffer"=w929, "refreshrate"=w928, "Vx-ref"=w935, "Vy-ref"=w937, "srate"=w926, "finite"=w939, "cont"=w938, "wavdet"=w940, "avpp"=w936, "srateAODO"=w933, "bufferAI"=w929, "bin"=w931, "Angle Img"=w923, "Vxminref"=w922, "Vxmaxref"=w921, "Vyminref"=w920, "Vymaxref"=w919, "Xpixels Img"=w918, "Ypixels Img"=w917, "Pel"=w915, "Vz-reset"=0.0, "AIoverride"=w913, "type"="Lifetime (contour)") -> (w941:T12)
                    n4084 = Reciprocal(x=w928) -> (1/x=w925:dbl)
                    n4085 = local write "refreshtime"(w925) -> ()
                    n4086 = call "2pparameters.vi"("Params in"=w941, "command"="set") -> ()  [unwired: 1 out]
                  }
                  frame "X-Y-Z-t movie" {
                  }
                  frame "linescan" {
                  }
                  frame "Timetrace" {
                    n4087 = local read "Vy-min draw"() -> (w953:dbl)
                    n4088 = local read "Vy-max draw"() -> (w952:dbl)
                    n4089 = local read "Vx-min draw"() -> (w955:dbl)
                    n4090 = local read "Vx-max draw"() -> (w954:dbl)
                    n4091 = local read "xpixels ref"() -> (w951:i32)
                    n4092 = local read "ypixels ref"() -> (w950:i32)
                    n4093 = local read "ROI Type"() -> (w949:u16)
                    n4094 = local read "srateAODOtt"() -> (w960:dbl)
                    n4095 = local read "# of frames"() -> (w965:i32)
                    n4096 = local read "refreshtime"() -> (w957:dbl)
                    n4097 = local read "Pel"() -> (w948:dbl)
                    n4098 = local read "bin"() -> (w963:dbl)
                    n4099 = local read "Override AI buffer"() -> (w946:bool)
                    n4100 = local read "finite samples"() -> (w972:bool)
                    n4101 = local read "srateAODOtt"() -> (w959:dbl)
                    n4102 = local read "srateAODOtt"() -> (w966:dbl)
                    n4103 = local read "continuous"() -> (w971:bool)
                    n4104 = local read "Angle ref"() -> (w956:dbl)
                    n4105 = local read "wavdet"() -> (w973:bool)
                    n4106 = local read "Vx-ref"() -> (w968:dbl)
                    n4107 = local read "Vy-ref"() -> (w970:dbl)
                    n4108 = local read "avpp"() -> (w969:i32)
                    n4109 = call "tt_timeandsamples.vi"("bin"=w963, "refreshtime"=w957, "srateAODOtt"=w960, "tot#ofsamples"=w965) -> ("refreshrate"=w961:dbl, "refreshbuffer"=w962:i32, "timetracecycles"=w967:i32)  [unwired: 5 in]
                    n4110 = local read "bin"() -> (w964:dbl)
                    n4111 = call "2pparameters.vi"("command"="get") -> ("params out"=w976:T12)  [unwired: 1 in]
                    n4112 = Bundle By Name(cluster=w976, "Drawing Mode"=w949, "measpoints"=w965, "tt_cycles"=w967, "refreshbuffer"=w962, "refreshrate"=w961, "Vx-ref"=w968, "Vy-ref"=w970, "srate"=w959, "finite"=w972, "cont"=w971, "wavdet"=w973, "avpp"=w969, "srateAODO"=w966, "bufferAI"=w962, "bin"=w964, "Angle Img"=w956, "Vxminref"=w955, "Vxmaxref"=w954, "Vyminref"=w953, "Vymaxref"=w952, "Xpixels Img"=w951, "Ypixels Img"=w950, "Pel"=w948, "Vz-reset"=0.0, "AIoverride"=w946, "type"="Timetrace") -> (w974:T12)
                    n4113 = Reciprocal(x=w961) -> (1/x=w958:dbl)
                    n4114 = local write "refreshtime"(w958) -> ()
                    n4115 = call "2pparameters.vi"("Params in"=w974, "command"="set") -> ()  [unwired: 1 out]
                  }
                  frame "Lifetime (point)" {
                  }
                }
              }
              frame #1 {
                w979 = FALSE ("wavdet")
                n4116 = call "2pparameters.vi"("command"="get") -> ("params out"=w983:T12)  [unwired: 1 in]
                n4117 = Bundle By Name(cluster=w983, "finite"=w979, "cont"=w979, "wavdet"=TRUE) -> (w980:T12)
                n4118 = call "2pparameters.vi"("Params in"=w980, "command"="set") -> ()  [unwired: 1 out]
              }
              frame #2 {
                n4119 = local read "DO channels"() -> (w988:u16)
                n4120 = call "2pparameters.vi"("command"="get") -> ("params out"=w990:T12)  [unwired: 1 in]
                n4121 = Unbundle By Name(w990) -> ("aDO"=w989:u32[])
                n4122 = Search 1D Array(1D array=w989, element=w988) -> (index of element=w986:i32)  [unwired: 1 in]
                n4123 = Greater?(x=w986, y=-1) -> (0:w985:bool)
                n4124 = case shown="True" w985 {
                  tunnel: w986 -> [_ w999]
                  frame False {
                  }
                  frame True {
                    n4125 = local read "Meastab"() -> (w993:enum32{"X-Y Image", "Linescan", "Timetrace"})
                    n4126 = local read "Digital padding value"() -> (w994:dbl)
                    n4127 = local read "Digital time offset (s)"() -> (w995:dbl)
                    n4128 = case shown="\"Timetrace\"" w993 {
                      tunnel: [w1000 w1001] -> w992
                      frame "X-Y Image", Default {
                        n4129 = local read "Sampling rate"() -> (w1000:dbl)
                      }
                      frame "Timetrace" {
                        n4130 = local read "srateAODOtt"() -> (w1001:dbl)
                      }
                    }
                    n4131 = local read "Digital Freq (Hz)"() -> (w997:dbl)
                    n4132 = local read "Digital phase (s)"() -> (w996:dbl)
                    n4133 = local read "Digital DC (%)"() -> (w998:dbl)
                    n4134 = call "replace DO wf param.vi"("Digital Freq (Hz)"=w997, "Digital DC (%)"=w998, "Digital phase"=w996, "Sampling frequency (Hz)"=w992, "Digital time offset (s)"=w995, "index of DO wave"=w999, "padding value"=w994) -> ()  [unwired: 4 in]
                  }
                }
              }
              frame #3 {
                n4135 = case shown="True" w1002 {
                  tunnel: w1003 -> [_ w1010]
                  frame False {
                  }
                  frame True {
                    n4136 = local read "Meastab"() -> (w1007:enum32{"X-Y Image", "Linescan", "Timetrace"})
                    n4137 = call "waveformparamsv2.vi"("command"="get") -> ("Params out"=w1026:T16)  [unwired: 4 in, 2 out]
                    n4138 = Unbundle By Name(w1026) -> ("DO parameters"=w1025:T19)
                    n4139 = property on="refwf" class="Ring (strict)"() -> ("RingText.Text"=w1032:string)  [unwired: 2 in, 2 out]
                    n4140 = case shown="\"Timetrace\"" w1007 {
                      tunnel: [w1033 w1034] -> w1006
                      frame "X-Y Image", Default {
                        n4141 = local read "Sampling rate"() -> (w1033:dbl)
                      }
                      frame "Timetrace" {
                        n4142 = local read "srateAODOtt"() -> (w1034:dbl)
                      }
                    }
                    n4143 = call "waveformsAObuffer.vi"("command"="get") -> ("AO wf out"=w1030:waveform(dbl)[])  [unwired: 1 in]
                    n4144 = call "waveformsDObuffer.vi"("command"="get") -> ("DO wf out"=w1028:digitalwaveform[])  [unwired: 1 in]
                    n4145 = call "referfencesize.vi"("Digital waveforms in"=w1028, "Analog waveforms in"=w1030, "reference waveforms to"=w1032) -> ("number of samples"=w1023:i32)  [unwired: 2 in]
                    n4146 = Index Array(array=w1025, index=w1010) -> (element=w1024:T20)
                    n4147 = call "waveformsDObuffer.vi"("command"="get") -> ("DO wf out"=w1020:digitalwaveform[])  [unwired: 1 in]
                    n4148 = call "simple digital from wf params.vi"("waveform params"=w1024, "number of samples"=w1023) -> ("digital waveform"=w1022:digitalwaveform)
                    n4149 = property on="refwf" class="Ring (strict)"() -> ("RingText.Text"=w1012:string)  [unwired: 2 in, 2 out]
                    n4150 = Replace Array Subset(array=w1020, new element=w1022, index=w1010) -> (w1011:digitalwaveform[])
                    n4151 = call "waveformsAObuffer.vi"("command"="get") -> ("AO wf out"=w1019:waveform(dbl)[])  [unwired: 1 in]
                    n4152 = local read "wavdet"() -> (w1009:bool)
                    n4153 = call "correctwaveformsizetemp.vi"("new sampling frequency (Hz)"=w1006, "start"=FALSE, "reference waveforms to"=w1012, "Analog waveforms in"=w1019, "stop"=FALSE, "Digital waveforms in"=w1011) -> ("analog wf out"=w1015:waveform(dbl)[], "Digital wf out"=w1013:digitalwaveform[], "measpoints"=w1008:i32)
                    n4154 = local write "Analog Lines Plot"(w1015) -> ()
                    n4155 = call "GetNumCamFramesv2.vi"("Digital Waveform Graph"=w1013) -> ("Numeric"=w1014:i32)  [unwired: 10 in]
                    n4156 = local write "Digital Lines Plot"(w1013) -> ()
                    n4157 = case shown="True" w1009 {
                      tunnel: w1008 -> [_ w1035]
                      frame False {
                      }
                      frame True {
                        n4158 = local write "# of frames"(w1035) -> ()
                      }
                    }
                    n4159 = call "waveformsAObuffer.vi"("AO wf in"=w1015, "command"="set") -> ()  [unwired: 1 out]
                    n4160 = call "waveformsDObuffer.vi"("DO wf in"=w1013, "command"="set") -> ()  [unwired: 1 out]
                    n4161 = local write "Total Camera Frames"(w1014) -> ()
                  }
                }
              }
              frame #4 {
                n4162 = local read "finite samples"() -> (w1036:bool)
                n4163 = local read "continuous"() -> (w1037:bool)
                n4164 = local read "wavdet"() -> (w1038:bool)
                n4165 = call "2pparameters.vi"("command"="get") -> ("params out"=w1041:T12)  [unwired: 1 in]
                n4166 = Bundle By Name(cluster=w1041, "finite"=w1036, "cont"=w1037, "wavdet"=w1038) -> (w1039:T12)
                n4167 = call "2pparameters.vi"("Params in"=w1039, "command"="set") -> ()  [unwired: 1 out]
              }
            }
          }
          event "refwf": Value Change {
            n4168 = event-data() -> ()  [unwired: 1 in, 6 out]
            n4169 = stacked-sequence {
              frame #0 {
                n4170 = local read "Measurement"() -> (w1043:T5)
                n4171 = case shown="\"X-Y-t movie\", Default" w1043 {
                  frame "X-Y-t movie", Default {
                    n4172 = local read "avpp"() -> (w1064:i32)
                    n4173 = local read "Angle ref"() -> (w1063:dbl)
                    n4174 = local read "ROI Type"() -> (w1062:u16)
                    n4175 = local read "xpixels ref"() -> (w1059:i32)
                    n4176 = local read "Vx-min ref"() -> (w1058:dbl)
                    n4177 = local read "Vx-max ref"() -> (w1057:dbl)
                    n4178 = local read "ypixels ref"() -> (w1055:i32)
                    n4179 = local read "Vy-min ref"() -> (w1056:dbl)
                    n4180 = local read "Vy-max ref"() -> (w1052:dbl)
                    n4181 = local read "Sampling rate"() -> (w1046:dbl)
                    n4182 = local read "finite samples"() -> (w1047:bool)
                    n4183 = local read "continuous"() -> (w1050:bool)
                    n4184 = local read "wavdet"() -> (w1051:bool)
                    n4185 = local read "# of frames"() -> (w1049:i32)
                    n4186 = local read "maxbufferAI"() -> (w1048:i32)
                    n4187 = local read "Override AI buffer"() -> (w1044:bool)
                    n4188 = call "2pparameters.vi"("command"="get") -> ("params out"=w1061:T12)  [unwired: 1 in]
                    n4189 = Bundle By Name(cluster=w1061, "type"="X-Y-t movie", "avpp"=w1064, "Angle Img"=w1063, "Xpixels Img"=w1059, "Vx-min Img"=w1058, "VX-max Img"=w1057, "Ypixels Img"=w1055, "Vy-min Img"=w1056, "Vy-max Img"=w1052, "srate"=w1046, "srate Img"=w1046, "finite"=w1047, "cont"=w1050, "wavdet"=w1051, "measpoints"=w1049, "maxbufferAI"=w1048, "Drawing Mode"=w1062, "Vz-reset"=0.0, "AIoverride"=w1044) -> (w1053:T12)
                    n4190 = call "2pparameters.vi"("Params in"=w1053, "command"="set") -> ()  [unwired: 1 out]
                  }
                  frame "X-Y-Z stack" {
                    n4191 = call "2pparameters.vi"("command"="get") -> ("params out"=w1068:T12)  [unwired: 1 in]
                    n4192 = Bundle By Name(cluster=w1068, "type"="X-Y-Z stack") -> (w1066:T12)
                    n4193 = call "2pparameters.vi"("Params in"=w1066, "command"="set") -> ()  [unwired: 1 out]
                  }
                  frame "Lifetime (scan)" {
                    n4194 = call "2pparameters.vi"("command"="get") -> ("params out"=w1073:T12)  [unwired: 1 in]
                    n4195 = Bundle By Name(cluster=w1073, "type"="Lifetime (scan)") -> (w1071:T12)
                    n4196 = call "2pparameters.vi"("Params in"=w1071, "command"="set") -> ()  [unwired: 1 out]
                  }
                  frame "Lifetime (contour)" {
                    n4197 = local read "Vy-min draw"() -> (w1083:dbl)
                    n4198 = local read "Vy-max draw"() -> (w1082:dbl)
                    n4199 = local read "Vx-min draw"() -> (w1085:dbl)
                    n4200 = local read "Vx-max draw"() -> (w1084:dbl)
                    n4201 = local read "xpixels ref"() -> (w1081:i32)
                    n4202 = local read "ypixels ref"() -> (w1080:i32)
                    n4203 = local read "ROI Type"() -> (w1079:u16)
                    n4204 = local read "srateAODOtt"() -> (w1090:dbl)
                    n4205 = local read "# of frames"() -> (w1095:i32)
                    n4206 = local read "refreshtime"() -> (w1087:dbl)
                    n4207 = local read "Pel"() -> (w1078:dbl)
                    n4208 = local read "bin"() -> (w1093:dbl)
                    n4209 = local read "Override AI buffer"() -> (w1076:bool)
                    n4210 = local read "finite samples"() -> (w1102:bool)
                    n4211 = local read "srateAODOtt"() -> (w1089:dbl)
                    n4212 = local read "srateAODOtt"() -> (w1096:dbl)
                    n4213 = local read "continuous"() -> (w1101:bool)
                    n4214 = local read "Angle ref"() -> (w1086:dbl)
                    n4215 = local read "wavdet"() -> (w1103:bool)
                    n4216 = local read "Vx-ref"() -> (w1098:dbl)
                    n4217 = local read "Vy-ref"() -> (w1100:dbl)
                    n4218 = local read "avpp"() -> (w1099:i32)
                    n4219 = call "tt_timeandsamples.vi"("bin"=w1093, "refreshtime"=w1087, "srateAODOtt"=w1090, "tot#ofsamples"=w1095) -> ("refreshrate"=w1091:dbl, "refreshbuffer"=w1092:i32, "timetracecycles"=w1097:i32)  [unwired: 5 in]
                    n4220 = local read "bin"() -> (w1094:dbl)
                    n4221 = call "2pparameters.vi"("command"="get") -> ("params out"=w1106:T12)  [unwired: 1 in]
